vi "check if at destination.vi"(8 "error in (no error)":errorcluster, 11 "focus in":refnum<class "focus.lvclass">) -> (0 "error out":errorcluster, 2 "at destination?":bool, 3 "focus out":refnum<class "focus.lvclass">)   [LabVIEW 2012, in "focus.lvclass"]
uses:
  focus.lvclass
  focus.lvclass/focus.ctl
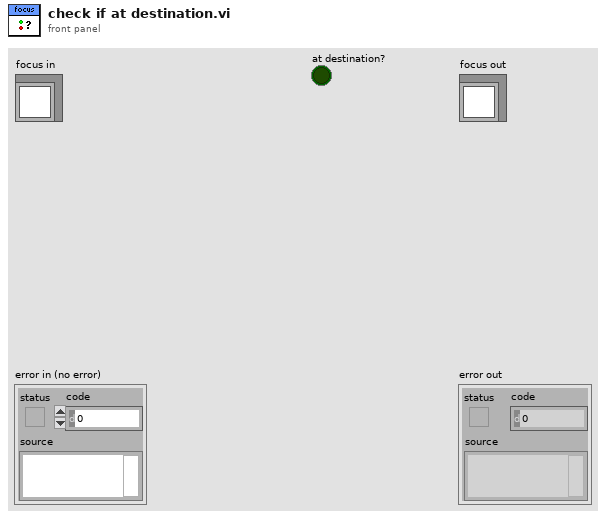
[diagram p1: front panel]
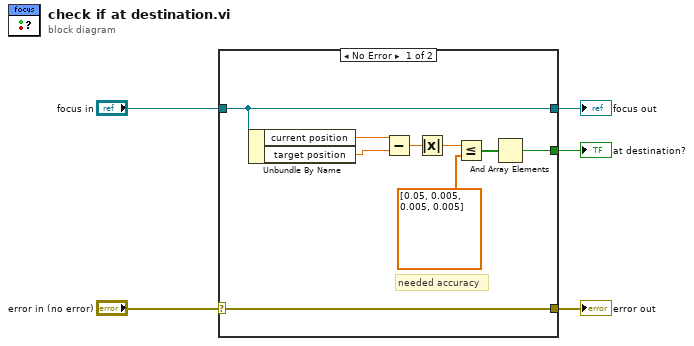
[diagram p0: block diagram]
diagram:
  n1 = case shown="No Error" "error in (no error)" {
    selector: "error in (no error)" -> [w14 w16]
    tunnel: [w14 w16] -> w4
    tunnel: [w13 w15] -> w2
    tunnel: "focus in" -> [w13 w15]
    tunnel: [w6 _] -> w1
    frame No Error {
      # "needed accuracy"
      n2 = Unbundle By Name(w13) -> ("current position"=w10:dbl, "target position"=w9:dbl)
      n3 = Subtract(x=w10, y=w9) -> (x-y=w11:dbl)
      n4 = Absolute Value(x=w11) -> (abs(x)=w12:dbl)
      n5 = Less Or Equal?(x=w12, y=dbl[] [0.05, 0.005, 0.005, 0.005]) -> (x <= y?=w7:bool[])
      n6 = And Array Elements(Boolean array=w7) -> (logical AND=w6:bool)
    }
    frame Error {
    }
  }
  "error out" <- w4
  "focus out" <- w2
  "at destination?" <- w1
